vi "set_instruments (SubVI).vi"(0 "process_list":T4, 2 "signal type":T2(ring), 4 "electrodes reference":refnum<vi>, 5 "instrument config":T3, 6 "Num samples":i32, 7 "small amp":dbl=1.0 format="%0.2p", 9 "Volt vs pos array":cluster{dbl, dbl}[](array[cluster]), 11 "small amp freq":dbl=10.0 format="%0.2p", 13 "Add small amp?":bool, 14 "encode_bits":bool[](array[boolean])) -> (17 "DC volts arr":dbl[](array[numeric]), 19 "instrument out":T1)   [LabVIEW 2018]
uses:
  <vilib>/DAQmx/write.llb/DAQmx Write (Analog 2D DBL NChan NSamp).vi
  <vilib>/DAQmx/miscellaneous.llb/DAQmx Fill In Error Info.vi
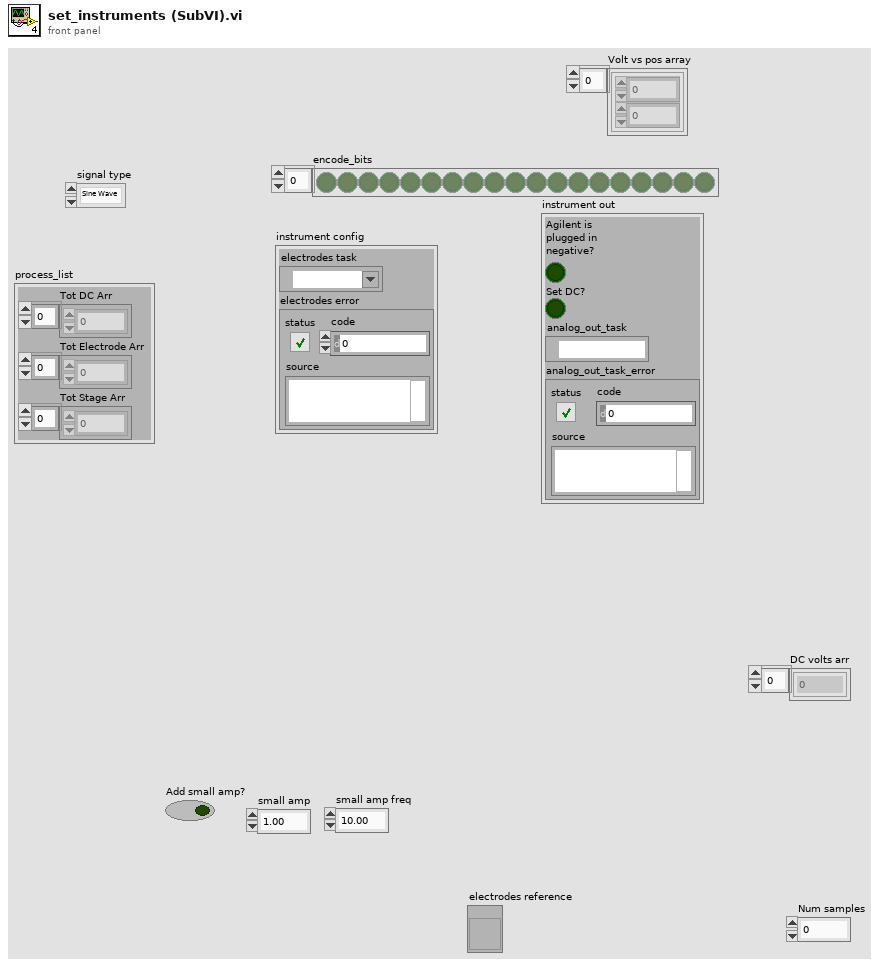
[diagram p1: front panel]
types:
  T1 = cluster{"Agilent is \nplugged in \nnegative?":bool, "Set DC?":bool, "analog_out_task":refnum<k21>, "analog_out_task_error":errorcluster}
  T2 = enum16{"Sine Wave", "Triangle Wave", "Square Wave", "Sawtooth Wave"}
  T3 = cluster{"electrodes task":refnum<k21>, "electrodes error":errorcluster}
  T4 = cluster{"Tot DC Arr":dbl[], "Tot Electrode Arr":dbl[], "Tot Stage Arr":dbl[]}
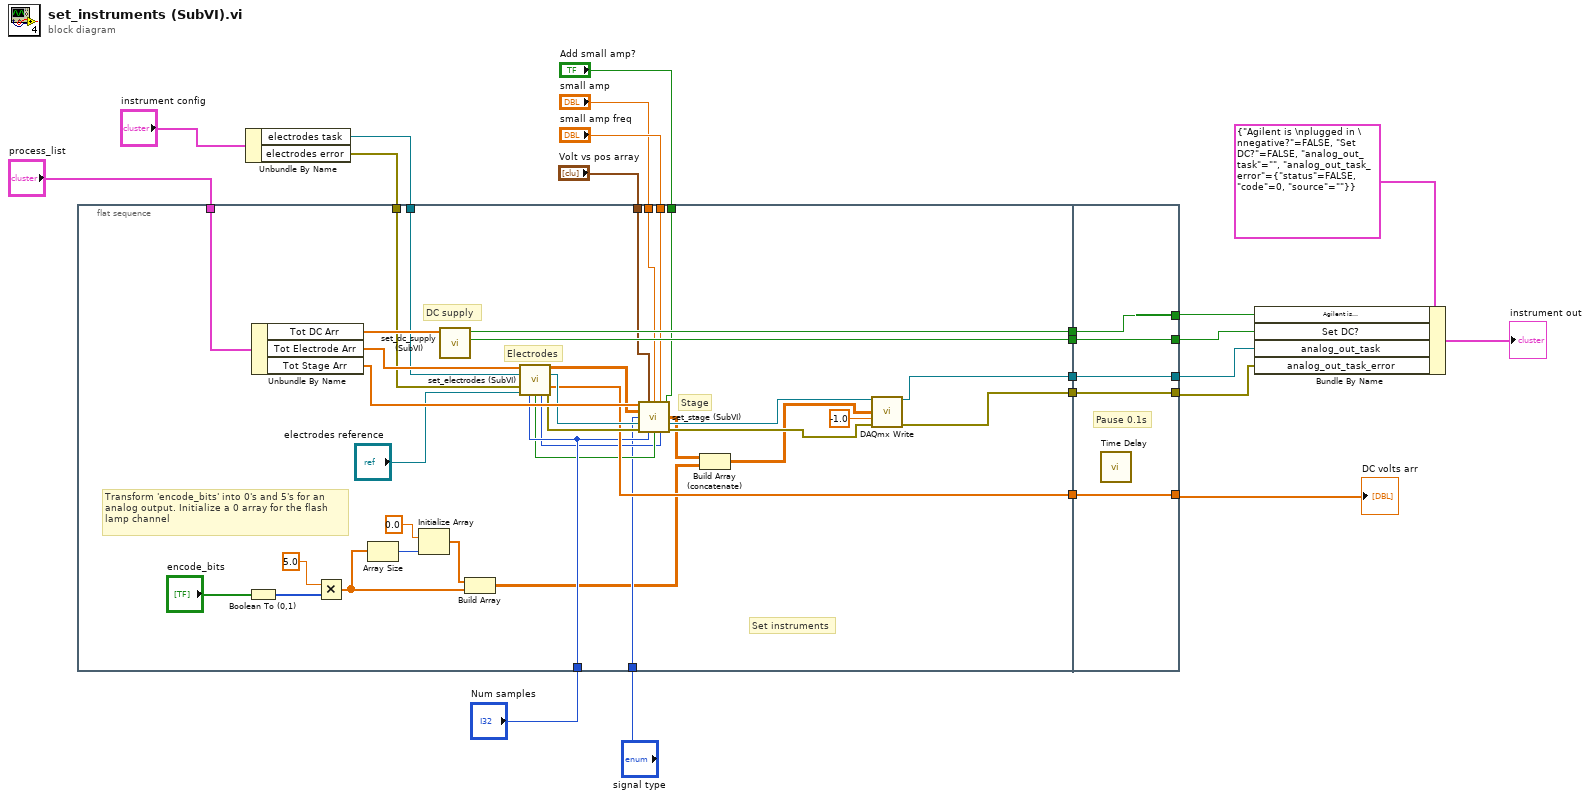
[diagram p0: block diagram]
diagram:
  n1 = flat-sequence {
    tunnel: "process_list" -> [w58]
    tunnel: w19 -> [w55]
    tunnel: w20 -> [w54]
    tunnel: [w31] -> w18
    tunnel: [w53] -> w17
    tunnel: [w30] -> w16
    tunnel: [w51] -> w15
    tunnel: [w46] -> w14
    tunnel: "Num samples" -> [w45]
    tunnel: "small amp freq" -> [w42]
    tunnel: "small amp" -> [w40]
    tunnel: "Add small amp?" -> [w41]
    tunnel: "Volt vs pos array" -> [w39]
    tunnel: "signal type" -> [w38]
    tunnel: [w61] -> w3
    tunnel: [w62] -> w6
    tunnel: [w63] -> w4
    tunnel: w18 -> [w63]
    tunnel: w17 -> [w62]
    tunnel: w16 -> [w61]
    tunnel: w15 -> [w60]
    tunnel: [w60] -> w5
    tunnel: [w59] -> w13
    tunnel: w14 -> [w59]
    frame #0 {
      # "Transform 'encode_bits' into 0's and 5's for an\nanalog output. Initialize a 0 array for the flash \nlamp channel"
      # "Stage"
      # "Electrodes"
      # "DC supply"
      # "Set instruments"
      n2 = Boolean To (0,1)(Boolean="encode_bits") -> (0, 1=w36:i16[])
      n3 = Unbundle By Name(w58) -> ("Tot DC Arr"=w57:dbl[], "Tot Electrode Arr"=w56:dbl[], "Tot Stage Arr"=w52:dbl[])
      n4 = Multiply(x=5.0 ("maximum value"), y=w36) -> (x*y=w23:dbl[])
      n5 = Array Size(array=w23) -> (size(s)=w28:i32)
      n6 = Initialize Array(0.0 ("maximum value"), w28) -> (w26:dbl[])
      n7 = call "set_dc_supply (SubVI).vi"("Tot DC Arr"=w57) -> ("Set DC?"=w51:bool, "Agilent is \nplugged in \nnegative?"=w53:bool)  [unwired: 9 in]
      n8 = Build Array(w26, w23) -> (w25:dbl[][])
      n9 = call "set_electrodes (SubVI).vi"("Tot Electrode Arr"=w56, "electrodes task 2"=w55, "electrodes error"=w54, "electrodes reference"="electrodes reference", "Num samples"=w45) -> ("electrode arr"=w50:dbl[][], "electrodes task"=w49:refnum<k21>, "DC volts arr"=w46:dbl[], "Use arbitrary\nforce func?"=w44:bool, "Electrode to sweep:"=w43:i32, "electrodes task error"=w48:errorcluster)  [unwired: 5 in]
      n10 = call "set_stage (SubVI).vi"("Tot Stage Arr"=w52, "Volt vs pos array"=w39, "small amp"=w40, "small amp freq"=w42, "Add small amp?"=w41, "electrode arr"=w50, "signal type"=w38, "electrodes task"=w49, "electrodes task error"=w48, "Num samples"=w45, "Use arb force?"=w44, "Electrode to sweep"=w43) -> ("electrode_stage_arr"=w29:dbl[][], "electrodes task 2"=w33:refnum<k21>, "electrodes task error 2"=w32:errorcluster)  [unwired: 1 in]
      n11 = Build Array (concatenate)(w29, w25) -> (w24:dbl[][])
      n12 = call-poly <vilib>:"DAQmx Write.vi"("task/channels in"=w33, "data"=w24, "timeout"=-1.0, "error in"=w32) -> ("task out"=w31:refnum<k21>, "error out"=w30:errorcluster)  [unwired: 9 in, 1 out]
    }
    frame #1 {
      # "Pause 0.1s"
      n13 = call "Time Delay"() -> ()  [unwired: 11 in, 1 out]
    }
  }
  n14 = Unbundle By Name("instrument config") -> ("electrodes task"=w19:refnum<k21>, "electrodes error"=w20:errorcluster)
  n15 = Bundle By Name(cluster=T1 {"Agilent is \nplugged in \nnegative?"=FALSE, "Set DC?"=FALSE, "analog_out_task"="", "analog_out_task_error"={"status"=FALSE, "code"=0, "source"=""}} ("input cluster"), "Agilent is \nplugged in \nnegative?"=w6, "Set DC?"=w5, "analog_out_task"=w4, "analog_out_task_error"=w3) -> (→"instrument out":T1)
  "DC volts arr" <- w13
